vi "Obtain Notifier.vi"(7 "Case":enum16{"Obtain", "Read"}(ring), 8 "error in (no error)":errorcluster) -> (0 "error out":errorcluster, 3 "notifiers out":T1)   [LabVIEW 2022 SP3]
uses:
  Controls/UI Data.ctl
  Controls/All Notifer.ctl
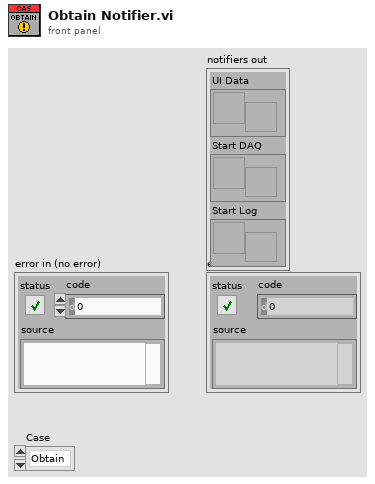
[diagram p1: front panel]
types:
  T1 = typedef "All Notifer.ctl" = cluster{"UI Data":refnum<notifier>, "Start DAQ":refnum<notifier>, "Start Log":refnum<notifier>}
  T2 = typedef "UI Data.ctl" = cluster{"Data":cluster{"AI":waveform(dbl)[], "DI":digitalwaveform[], "TC":waveform(dbl)[]}}
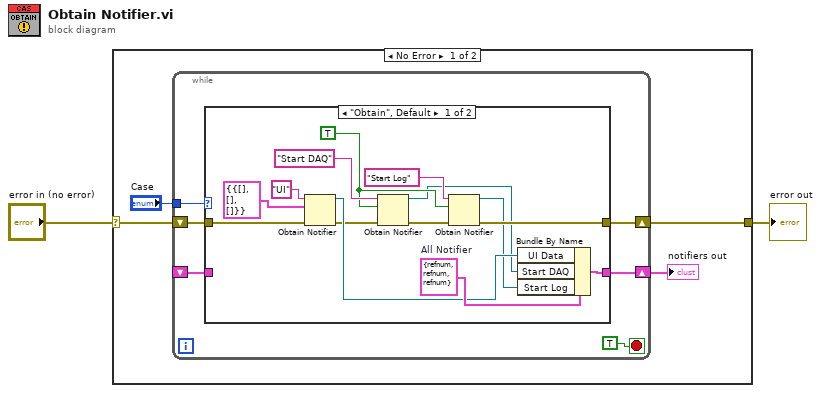
[diagram p0: block diagram]
diagram:
  n1 = case shown="No Error" "error in (no error)" {
    selector: "error in (no error)" -> [w6 w29]
    tunnel: [w5 w29] -> w1
    frame No Error {
      n2 = while {
        shift-right: [w11] -> w5
        shift-left: w6 -> [w12]
        tunnel: "Case" -> [w9]
        shift-right: [w8] -> w3
        shift-left: _ -> [w7]
        stop <- TRUE stop-if-true
        n3 = case shown="\"Obtain\", Default" w9 {
          tunnel: w12 -> [w24 w27]
          tunnel: [w17 w27] -> w11
          tunnel: [w19 w28] -> w8
          tunnel: w7 -> [_ w28]
          frame "Obtain", Default {
            w23 = T1 {"UI Data"=refnum, "Start DAQ"=refnum, "Start Log"=refnum}  # All Notifier
            w15 = TRUE ("create if not found? (T)")
            n4 = Obtain Notifier(name (unnamed)="UI", notification data type=T2 {"Data"={"AI"=[], "DI"=[], "TC"=[]}} ("UI Data"), error in (no error)=w24) -> (notifier out=w22:refnum<notifier>, error out=w20:errorcluster)  [unwired: 1 in, 1 out]
            n5 = Obtain Notifier(name (unnamed)="Start DAQ", notification data type=w15, error in (no error)=w20) -> (notifier out=w14:refnum<notifier>, error out=w18:errorcluster)  [unwired: 1 in, 1 out]
            n6 = Obtain Notifier(name (unnamed)="Start Log", notification data type=w15, error in (no error)=w18) -> (notifier out=w13:refnum<notifier>, error out=w17:errorcluster)  [unwired: 1 in, 1 out]
            n7 = Bundle By Name(cluster=w23, "UI Data"=w22, "Start DAQ"=w14, "Start Log"=w13) -> (w19:T1)
          }
          frame "Read" {
          }
        }
      }
      "notifiers out" <- w3
    }
    frame Error {
    }
  }
  "error out" <- w1
